vi "Translator.FormatEnumSrc.vi"(0 "text in":string, 1 "quotas?(T)":bool=TRUE) -> (2 "text out":string)   [LabVIEW 2019, in "Tools.lvlib"]
uses:
  Tools.lvlib
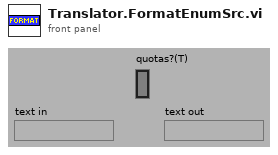
[diagram p1: front panel]
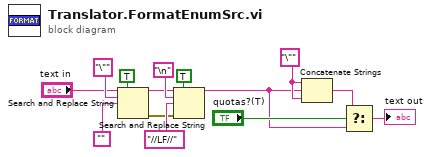
[diagram p0: block diagram]
diagram:
  w8 = "\""
  n1 = Search and Replace String(replace all?=TRUE ("replace all? (F)"), input string="text in", search string="\"", replace string="") -> (result string=w6:string, error out=w7:errorcluster)  [unwired: 4 in, 2 out]
  n2 = Search and Replace String(replace all?=TRUE ("replace all? (F)"), input string=w6, search string="\n", replace string="//LF//" ("search string"), error in=w7) -> (result string=w3:string)  [unwired: 6 out]
  n3 = Concatenate Strings(w8, w3, w8) -> (w4:string)
  n4 = Select(t=w4, s="quotas?(T)", f=w3) -> (s? t:f=→"text out":string)
